vi "Pre-Build Custom Action TC.vi"(10 "Variant":variant) -> (0 "error out":errorcluster)   [LabVIEW 2019]
uses:
  <vilib>/Utility/traverseref.llb/TRef TravTarget.ctl
  <vilib>/Utility/traverseref.llb/VI Scripting - Traverse.lvlib
  <vilib>/LabVIEW Open Source Project/Unicity/RandomStringGenerator/RandomStringGenerator.lvclass
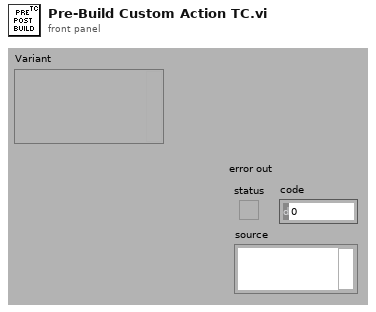
[diagram p1: front panel]
types:
  T1 = typedef "TRef TravTarget.ctl" = enum16{"FP", "BD", "Other"}
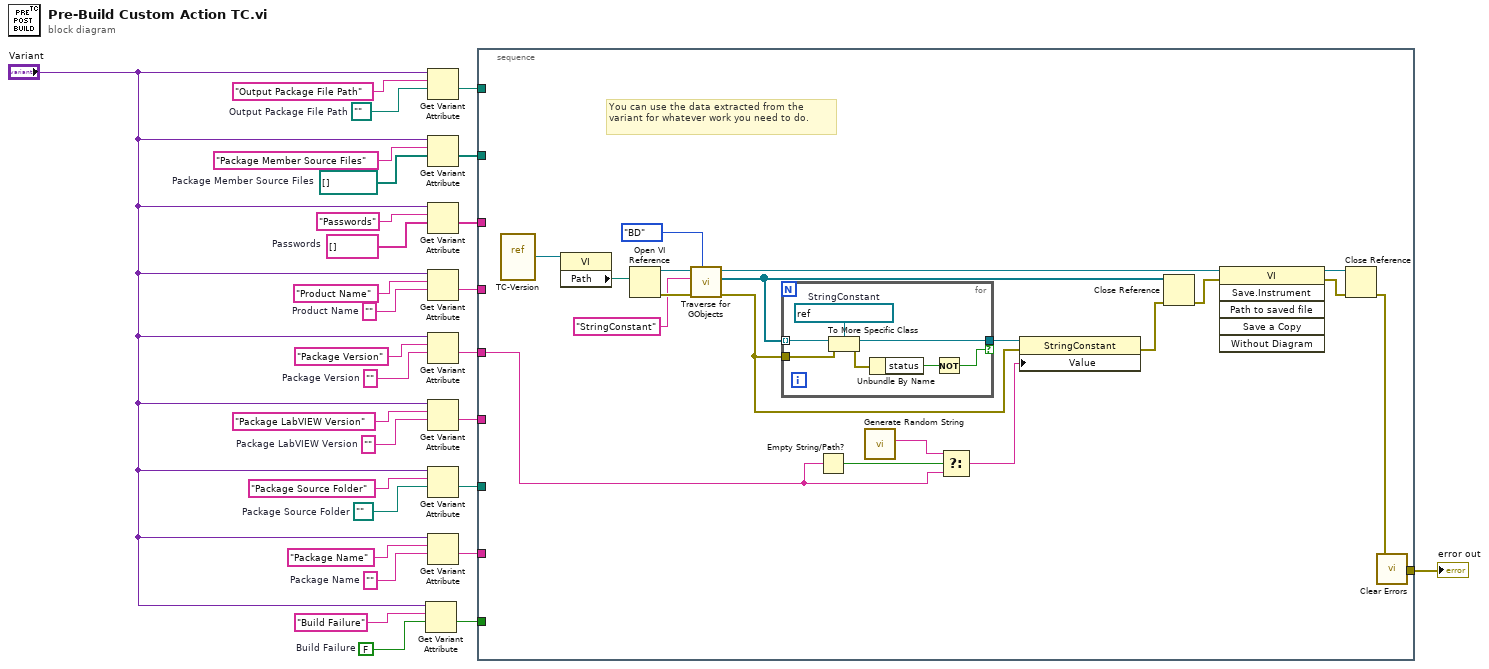
[diagram p0: block diagram]
diagram:
  w4 = FALSE  # Build Failure
  w14 = path ""  # Package Source Folder
  w15 = ""  # Package Name
  w18 = ""  # Package LabVIEW Version
  w20 = ""  # Package Version
  w22 = ""  # Product Name
  w24 = string[] []  # Passwords
  w26 = path[] []  # Package Member Source Files
  w28 = path ""  # Output Package File Path
  n1 = Get Variant Attribute(Variant="Variant", name="Build Failure", default value (empty Variant)=w4) -> (value=w2:bool)  [unwired: 1 in, 3 out]
  n2 = Get Variant Attribute(Variant="Variant", name="Output Package File Path", default value (empty Variant)=w28) -> (value=w13:path)  [unwired: 1 in, 3 out]
  n3 = Get Variant Attribute(Variant="Variant", name="Package Member Source Files", default value (empty Variant)=w26) -> (value=w12:path[])  [unwired: 1 in, 3 out]
  n4 = Get Variant Attribute(Variant="Variant", name="Passwords", default value (empty Variant)=w24) -> (value=w11:string[])  [unwired: 1 in, 3 out]
  n5 = Get Variant Attribute(Variant="Variant", name="Product Name", default value (empty Variant)=w22) -> (value=w10:string)  [unwired: 1 in, 3 out]
  n6 = Get Variant Attribute(Variant="Variant", name="Package Version", default value (empty Variant)=w20) -> (value=w9:string)  [unwired: 1 in, 3 out]
  n7 = Get Variant Attribute(Variant="Variant", name="Package LabVIEW Version", default value (empty Variant)=w18) -> (value=w8:string)  [unwired: 1 in, 3 out]
  n8 = Get Variant Attribute(Variant="Variant", name="Package Source Folder", default value (empty Variant)=w14) -> (value=w7:path)  [unwired: 1 in, 3 out]
  n9 = Get Variant Attribute(Variant="Variant", name="Package Name", default value (empty Variant)=w15) -> (value=w6:string)  [unwired: 1 in, 3 out]
  n10 = stacked-sequence {
    tunnel: w13 -> [_]
    tunnel: w12 -> [_]
    tunnel: w11 -> [_]
    tunnel: w10 -> [_]
    tunnel: w9 -> [w34]
    tunnel: w8 -> [_]
    tunnel: w7 -> [_]
    tunnel: w6 -> [_]
    tunnel: w2 -> [_]
    tunnel: [w30] -> w1
    frame #0 {
      # "You can use the data extracted from the variant for whatever work you need to do."
      n11 = vi-ref "TC-Version.vi"() -> (w44:refnum<vi>)
      n12 = property class="VI"(reference=w44) -> ("Path"=w45:path)  [unwired: 1 in, 2 out]
      n13 = Open VI Reference(vi path=w45) -> (vi reference=w39:refnum<vi>, error out=w41:errorcluster)  [unwired: 5 in]
      n14 = call <vilib>:"Traverse for GObjects.vi"("Traverse Target"=TRef_TravTarget."BD", "error in (no error)"=w41, "Class Name"="StringConstant", "VI Refnum"=w39) -> ("error out"=w43:errorcluster, "References"=w42:refnum<vi>[], "dup VI Refnum"=w46:refnum<vi>)  [unwired: 4 in, 1 out]
      n15 = for {
        tunnel: w42 -> [w56] mode=indexing
        tunnel: [w55] -> w40 if=w52
        tunnel: w43 -> [w54]
        w51 = refnum<vi> refnum  # StringConstant
        n16 = To More Specific Class(target class=w51, reference=w56, error in=w54) -> (specific class reference=w55:refnum<vi>, error out=w50:errorcluster)
        n17 = Unbundle By Name(w50) -> ("status"=w53:bool)
        n18 = Not(x=w53) -> (.not. x?=w52:bool)
      }
      n19 = Empty String/Path?(string/path=w34) -> (empty?=w35:bool)
      n20 = call <vilib>:"Generate Random String.vi"() -> ("Random String"=w32:string)  [unwired: 11 in]
      n21 = Select(t=w32, s=w35, f=w34) -> (s? t:f=w33:string)
      n22 = property on="Property Node" class="StringConstant"(reference=w40, error in=w43, "Value"=w33) -> (error out=w38:errorcluster)  [unwired: 1 out]
      n23 = Close Reference(reference=w42, error in (no error)=w38) -> (error out=w48:errorcluster)
      n24 = invoke class="VI" method="Save.Instrument"(reference=w46, error in=w48) -> (reference out=w47:refnum<vi>, error out=w49:errorcluster)  [unwired: 4 in, 4 out]
      n25 = Close Reference(reference=w47, error in (no error)=w49) -> (error out=w36:errorcluster)
      n26 = call <vilib>:"Clear Errors.vi"("error in (no error)"=w36) -> ("error out"=w30:errorcluster)  [unwired: 5 in, 1 out]
    }
  }
  "error out" <- w1
